vi "Shutter.vi"() -> ()   [LabVIEW 2014]
panel:
  in  "OK Button":bool
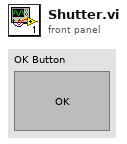
[diagram p1: front panel]
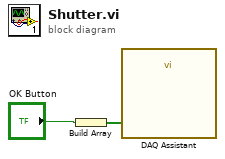
[diagram p0: block diagram]
diagram:
  n1 = Build Array("OK Button") -> (w2:bool[])
  n2 = call "DAQ Assistant"("data"=w2) -> ()  [unwired: 17 in, 2 out]
